vi "Convert BIN to TXT File.vi"(8 "error in (no error)":errorcluster, 11 "path":path) -> (0 "error out":errorcluster, 2 "Status":string)   [LabVIEW 2019, in "CAN Stream Support Workspace Shared.lvlib"]
uses:
  CAN Stream Support Workspace Shared.lvlib
  <vilib>/xnet/xnet.llb/XNET Frame CAN.ctl
  <vilib>/xnet/xnet.llb/XNET Frame Type CAN.ctl
  <vilib>/dlg_ctls.llb/Space Constant.vi
  <vilib>/Utility/error.llb/Trim Whitespace.vi
  Convert Time to UTC String.vi
  <vilib>/Utility/error.llb/Trim Whitespace One-Sided.vi
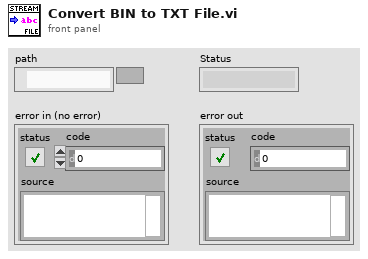
[diagram p1: front panel]
types:
  T1 = typedef "XNET Frame CAN.ctl" = cluster{"timestamp":timestamp, "payload":u8[], "identifier":u32, "type":T2, "extended?":bool, "echo?":bool}
  T2 = typedef "XNET Frame Type CAN.ctl" = u8
  T3 = enum16{"open", "replace", "create", "open or create", "replace or create", "replace or create with confirmation"}
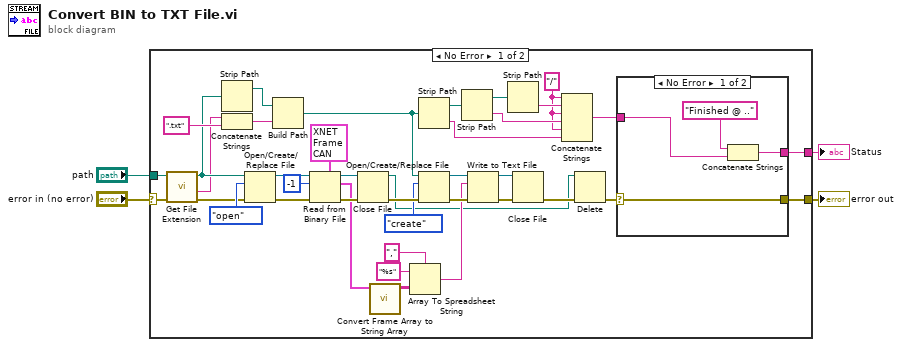
[diagram p0: block diagram]
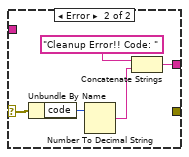
[diagram p2: hidden frame]
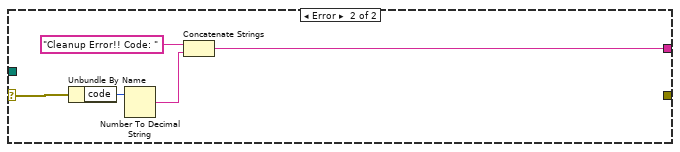
[diagram p3: hidden frame]
diagram:
  n1 = case shown="No Error" "error in (no error)" {
    selector: "error in (no error)" -> [w26 w55]
    tunnel: "path" -> [w32 _]
    tunnel: [w23 _] -> w2
    tunnel: [w24 w53] -> w4
    frame No Error {
      w6 = "/" ("string")
      n2 = call <vilib>:"Get File Extension.vi"("error in (no error)"=w26, "file"=w32) -> ("error out"=w27:errorcluster, "filename without extension"=w25:string, "dup file"=w28:path)  [unwired: 5 in, 2 out]
      n3 = Strip Path(path=w28) -> (stripped path=w13:path)  [unwired: 1 out]
      n4 = Concatenate Strings(w25, ".txt" ("string")) -> (w30:string)
      n5 = Open/Create/Replace File(file path (use dialog)=w28, error in=w27, operation (0:open)=T3."open") -> (refnum out=w41:refnum<file>, error out=w42:errorcluster)  [unwired: 3 in, 1 out]
      n6 = Build Path(base path=w13, name or relative path=w30) -> (appended path=w12:path)
      n7 = Read from Binary File(5:T1 {"timestamp"=timestamp(0 s since 1904-01-01), "payload"=[], "identifier"=0, "type"=0, "extended?"=FALSE, "echo?"=FALSE} ("CAN frame"), 8:w42, 10:-1 ("count (1)"), 11:w41) -> (0:w35:errorcluster, 2:w17:T1[], 3:w33:refnum<file>)  [unwired: 2 in, 1 out]
      n8 = Close File(refnum=w33, error in=w35) -> (path=w14:path, error out=w34:errorcluster)
      n9 = call "Convert Frame Array to String Array.vi"("Array in"=w17) -> ("Array out"=w21:string[][])  [unwired: 10 in]
      n10 = Array To Spreadsheet String(delimiter (Tab)=",", array=w21, 3:"%s" ("format string")) -> (spreadsheet string=w18:string)
      n11 = Strip Path(path=w12) -> (stripped path=w11:path, name=w7:string)
      n12 = Open/Create/Replace File(file path (use dialog)=w12, error in=w34, operation (0:open)=T3."create") -> (refnum out=w39:refnum<file>, error out=w38:errorcluster)  [unwired: 3 in, 1 out]
      n13 = Strip Path(path=w11) -> (stripped path=w10:path, name=w8:string)
      n14 = Write to Text File(file (use dialog)=w39, text=w18, error in=w38) -> (refnum out=w37:refnum<file>, error out=w36:errorcluster)  [unwired: 1 in, 1 out]
      n15 = Strip Path(path=w10) -> (name=w9:string)  [unwired: 1 out]
      n16 = Close File(refnum=w37, error in=w36) -> (error out=w16:errorcluster)  [unwired: 1 out]
      n17 = Concatenate Strings(w6, w9, w6, w8, w6, w7) -> (w5:string)
      n18 = Delete(path (use dialog)=w14, error in=w16) -> (error out=w15:errorcluster)  [unwired: 3 in, 2 out]
      n19 = case shown="No Error" w15 {
        selector: w15 -> [w45 w49]
        tunnel: [w46 w48] -> w24
        tunnel: [w45 _] -> w23
        tunnel: w5 -> [w44 _]
        frame No Error {
          n20 = Concatenate Strings("Finished @ .." ("string"), w44) -> (w46:string)
        }
        frame Error {
          n21 = Unbundle By Name(w49) -> ("code"=w51:i32)
          n22 = Number To Decimal String(number=w51) -> (decimal integer string=w52:string)  [unwired: 1 in]
          n23 = Concatenate Strings("Cleanup Error!! Code: ", w52) -> (w48:string)
        }
      }
    }
    frame Error {
      n24 = Unbundle By Name(w55) -> ("code"=w57:i32)
      n25 = Number To Decimal String(number=w57) -> (decimal integer string=w56:string)  [unwired: 1 in]
      n26 = Concatenate Strings("Cleanup Error!! Code: ", w56) -> (w53:string)
    }
  }
  "Status" <- w4
  "error out" <- w2
